vi "UpdatedEnumControls.vi"(7 "Seasons":T3(ring)=enum."Fall", 10 "Months":T1(ring)=enum."November", 11 "Colors":T2(ring)=enum."Red") -> ()   [LabVIEW 2012]
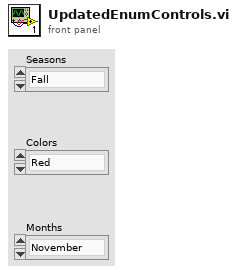
[diagram p1: front panel]
types:
  T1 = enum32{"LeapFeb", "January", "February", "March", "April", "May", "June", "July", "August", "September", "October", "November", "December"}
  T2 = enum16{"Crimson", "Red", "Green", "Blue", "Yellow", "Purple", "Orange"}
  T3 = enum32{"Rainy", "Fall", "Winter", "Spring", "Summer"}
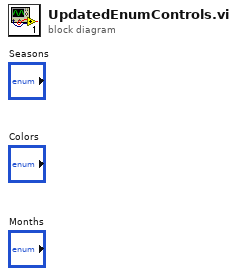
[diagram p0: block diagram]
diagram:
